vi "Parse Fields.vi"(8 "error in (no error)":errorcluster, 11 "URI in":refnum<class "URI.lvclass">) -> (0 "error out":errorcluster, 3 "URI out":refnum<class "URI.lvclass">)   [LabVIEW 2020, in "IO.lvlib" / "URI.lvclass"]
uses:
  URI.lvclass
  URI.lvclass/URI.ctl
  <vilib>/regexp/Match Regular Expression.xnode
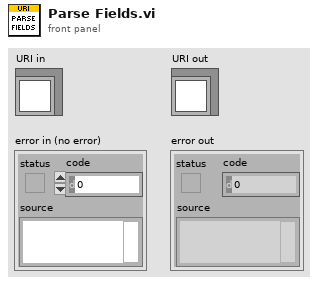
[diagram p1: front panel]
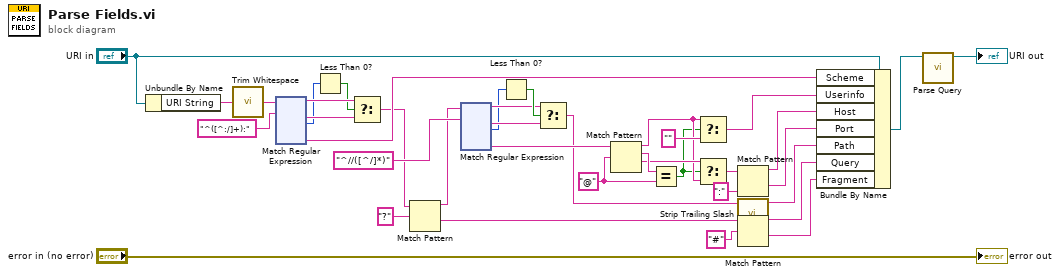
[diagram p0: block diagram]
diagram:
  w17 = "@" ("regular expression")
  n1 = Unbundle By Name("URI in") -> ("URI String"=w29:string)
  n2 = call <vilib>:"Trim Whitespace.vi"("string"=w29) -> ("trimmed string"=w24:string)  [unwired: 1 in]
  n3 = xnode "Match Regular Expression"("input string"=w24, "regular expression"="^([^:/]+):") -> ("before match"=w28:string, "after match"=w27:string, "offset past match"=w26:i32, "submatch 1"=w30:string)  [unwired: 4 in, 2 out]
  n4 = Less Than 0?(x=w26) -> (x < 0?=w25:bool)
  n5 = Select(t=w28, s=w25, f=w27) -> (s? t:f=w4:string)
  n6 = Match Pattern(string=w4, regular expression="?") -> (before substring=w3:string, after substring=w6:string)  [unwired: 1 in, 2 out]
  n7 = xnode "Match Regular Expression"("input string"=w3, "regular expression"="^//([^/]*)") -> ("before match"=w20:string, "after match"=w19:string, "offset past match"=w18:i32, "submatch 1"=w9:string)  [unwired: 4 in, 2 out]
  n8 = Less Than 0?(x=w18) -> (x < 0?=w21:bool)
  n9 = Select(t=w20, s=w21, f=w19) -> (s? t:f=w2:string)
  n10 = Match Pattern(string=w9, regular expression=w17) -> (before substring=w13:string, match substring=w16:string, after substring=w14:string)  [unwired: 1 in, 1 out]
  n11 = Equal?(x=w16, y=w17) -> (x = y?=w12:bool)
  n12 = Select(t=w13, s=w12, f="") -> (s? t:f=w36:string)
  n13 = Select(t=w14, s=w12, f=w13) -> (s? t:f=w11:string)
  n14 = Match Pattern(string=w11, regular expression=":") -> (before substring=w35:string, after substring=w34:string)  [unwired: 1 in, 2 out]
  n15 = call "Strip Trailing Slash.vi"("Path in"=w2) -> ("Path out"=w1:string)  [unwired: 10 in]
  n16 = Match Pattern(string=w6, regular expression="#") -> (before substring=w5:string, after substring=w31:string)  [unwired: 1 in, 2 out]
  n17 = Bundle By Name(cluster="URI in", "Scheme"=w30, "Userinfo"=w36, "Host"=w35, "Port"=w34, "Path"=w1, "Query"=w5, "Fragment"=w31) -> (w7:refnum<class "URI.lvclass">)
  n18 = call "Parse Query.vi"("URI in"=w7) -> ("URI out"=→"URI out":refnum<class "URI.lvclass">)  [unwired: 9 in, 1 out]
  "error out" <- "error in (no error)"
